vi "Query-Error.vi"(3 "error in (no error)":errorcluster, 4 "Input channel":T1, 5 "VISA resource name":refnum<visa-resource-name>) -> (0 "error out":errorcluster, 1 "Error Signal / V":dbl, 2 "VISA resource name out":refnum<visa-resource-name>)   [LabVIEW 2014, in "YbTempCtrl.lvlib"]
doc: "Performs an instrument error query before terminating the software connection to the instrument."
uses:
  YbTempCtrl.lvlib
  Typedefs/InputChannelTypedef.ctl
panel:
  out "read buffer":string
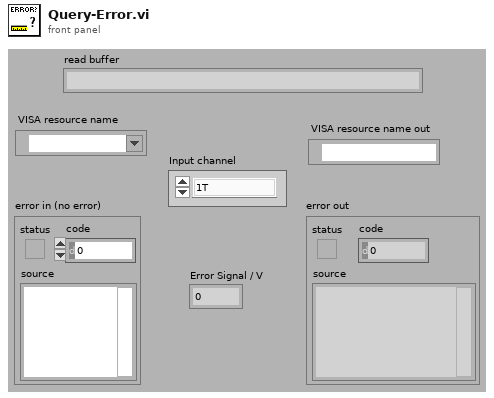
[diagram p1: front panel]
types:
  T1 = typedef "YbTempCtrl.lvlib/InputChannelTypedef.ctl" = enum16{"1T", "1V", "2T", "2V", "TMP", "POW"}
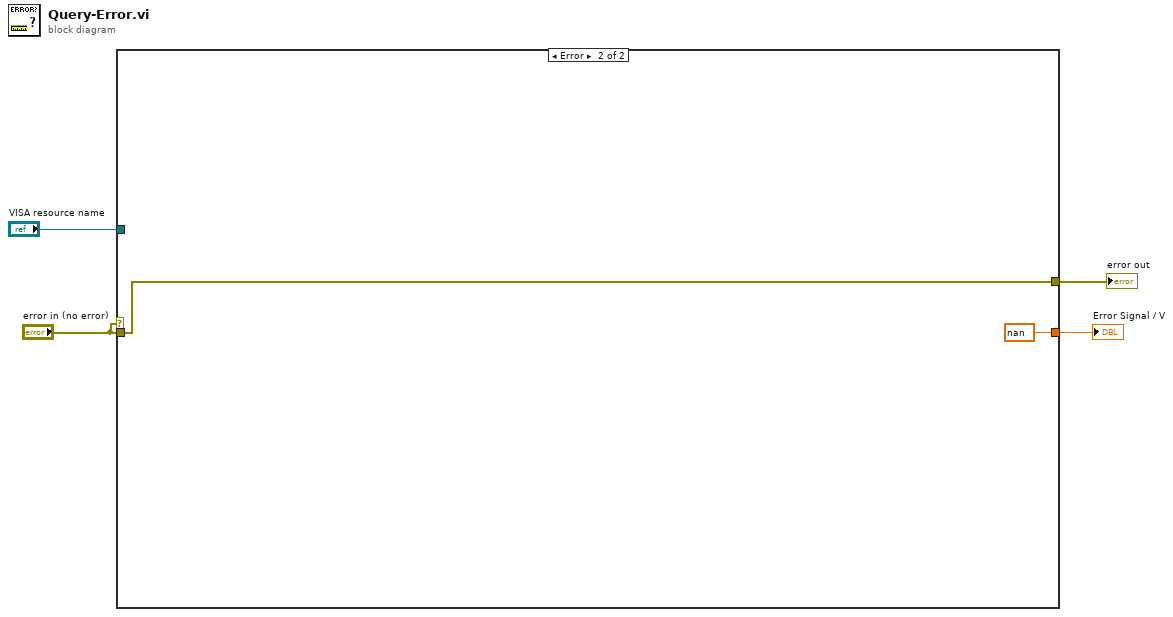
[diagram p0: block diagram]
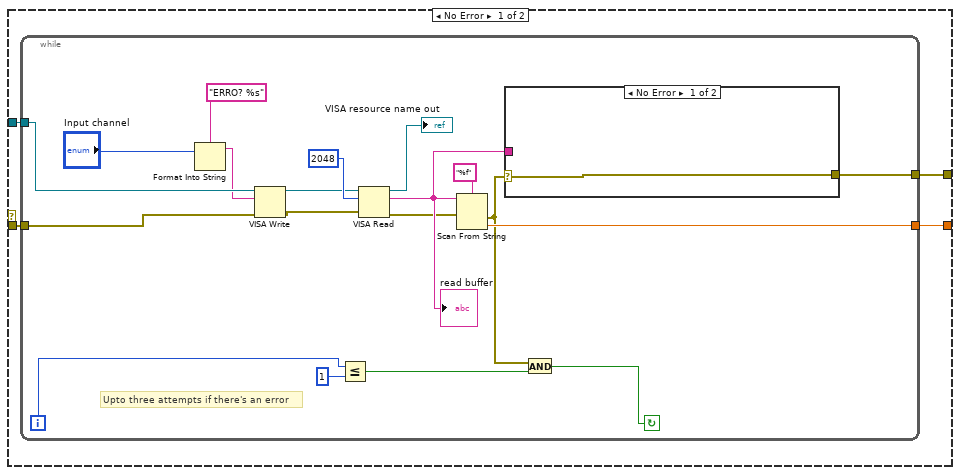
[diagram p2: hidden frame]
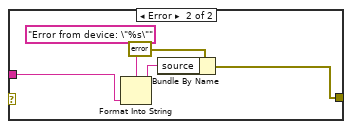
[diagram p3: hidden frame]
diagram:
  n1 = case shown="Error" "error in (no error)" {
    tunnel: "VISA resource name" -> [w8 _]
    tunnel: "error in (no error)" -> [w7 w35]
    tunnel: [w6 nan] -> w3
    tunnel: [w5 w35] -> w2
    frame No Error {
      n2 = while {
        tunnel: w8 -> [w27]
        tunnel: w7 -> [w25]
        tunnel: [w13] -> w6
        tunnel: [w12] -> w5
        i -> [w19]
        stop <- w20 continue-if-true
        # "Upto three attempts if there's an error"
        n3 = Format Into String(format string="ERRO? %s", "Input channel") -> (resulting string=w15:string)  [unwired: 2 in, 1 out]
        n4 = VISA Write(VISA resource name=w27, write buffer=w15, error in (no error)=w25) -> (VISA resource name out=w17:refnum<visa-resource-name>, error out=w18:errorcluster)  [unwired: 1 out]
        n5 = Less Or Equal?(x=w19, y=1) -> (x <= y?=w22:bool)
        n6 = VISA Read(VISA resource name=w17, byte count=u32 2048, error in (no error)=w18) -> (VISA resource name out=→"VISA resource name out":refnum<visa-resource-name>, read buffer=w11:string, error out=w10:errorcluster)  [unwired: 1 out]
        "read buffer" <- w11
        n7 = Scan From String(format string="%f", input string=w11, error in=w10) -> (error out=w9:errorcluster, output 1=w13:dbl)  [unwired: 2 in, 2 out]
        n8 = case shown="No Error" w9 {
          selector: w9 -> [w28 _]
          tunnel: [w28 w32] -> w12
          tunnel: w11 -> [_ w31]
          frame No Error {
          }
          frame Error {
            n9 = Format Into String(format string="Error from device: \"%s\"", w31) -> (resulting string=w30:string)  [unwired: 2 in, 1 out]
            n10 = Bundle By Name(cluster=errorcluster {"status"=TRUE, "code"=9999, "source"=""} ("error constant"), "source"=w30) -> (w32:errorcluster)
          }
        }
        n11 = And(x=w9, y=w22) -> (x .and. y?=w20:bool)
      }
    }
    frame Error {
    }
  }
  "Error Signal / V" <- w3
  "error out" <- w2
